vi "Create Error Object.vi"(8 "error in (no error)":errorcluster) -> (0 "error out":errorcluster, 2 "error":T1)   [LabVIEW 2019, in "JSON-RPC.lvlib"]
uses:
  JSON-RPC.lvlib
  typedefs/Error--Cluster.ctl
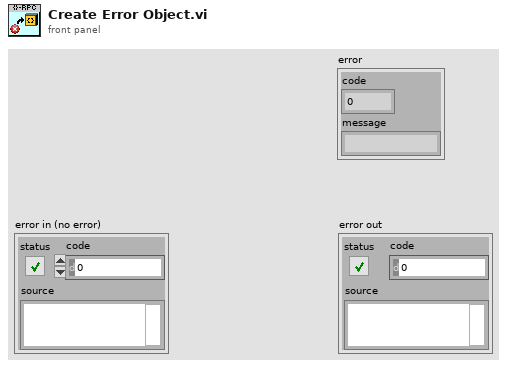
[diagram p1: front panel]
types:
  T1 = typedef "JSON-RPC.lvlib/Error--Cluster.ctl" = cluster{"code":i32, "message":string}
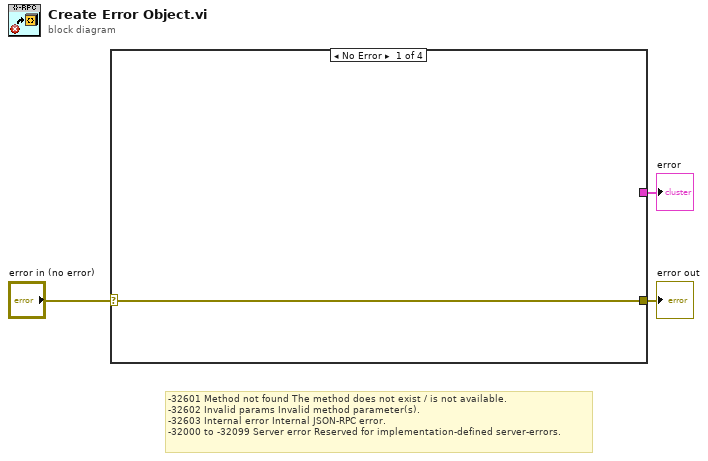
[diagram p0: block diagram]
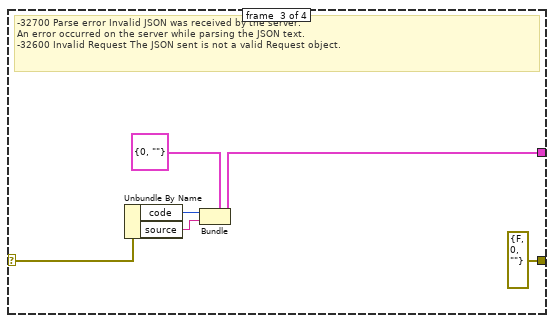
[diagram p3: hidden frame]
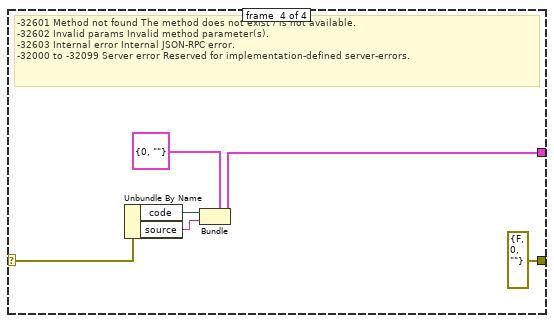
[diagram p4: hidden frame]
diagram:
  # "-32601\tMethod not found\tThe method does not exist / is not available.\n-32602\tInvalid params\tInvalid method parameter(s).\n-32603\tInternal error\tInternal JSON-RPC error.\n-32000 to -32099\tServer error\tReserved for implementation-defined server-errors."
  n1 = case shown="No Error" "error in (no error)" {
    selector: "error in (no error)" -> [w4 w5 w8 w14]
    tunnel: [w4 w5 errorcluster {"status"=FALSE, "code"=0, "source"=""} ("error IO") errorcluster {"status"=FALSE, "code"=0, "source"=""} ("error IO")] -> w2
    tunnel: [_ _ w6 w12] -> w1
    frame #0 {
    }
    frame #1 {
    }
    frame #2 {
      # "-32700\tParse error\tInvalid JSON was received by the server.\nAn error occurred on the server while parsing the JSON text.\n-32600\tInvalid Request\tThe JSON sent is not a valid Request object."
      n2 = Unbundle By Name(w8) -> ("code"=w11:i32, "source"=w10:string)
      n3 = Bundle(cluster=T1 {"code"=0, "message"=""} ("error"), "code"=w11, "message"=w10) -> (w6:T1)
    }
    frame #3 {
      # "-32601\tMethod not found\tThe method does not exist / is not available.\n-32602\tInvalid params\tInvalid method parameter(s).\n-32603\tInternal error\tInternal JSON-RPC error.\n-32000 to -32099\tServer error\tReserved for implementation-defined server-errors."
      n4 = Unbundle By Name(w14) -> ("code"=w17:i32, "source"=w16:string)
      n5 = Bundle(cluster=T1 {"code"=0, "message"=""} ("error"), "code"=w17, "message"=w16) -> (w12:T1)
    }
  }
  "error out" <- w2
  "error" <- w1
